vi "WAPIGetBoardType.vi"(9 "error in (no error)":errorcluster) -> (2 "Board Type":u32, 6 "error out":errorcluster)   [LabVIEW 2009]
uses:
  win50032.dll
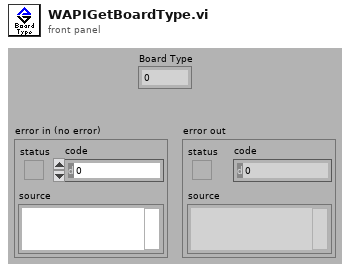
[diagram p1: front panel]
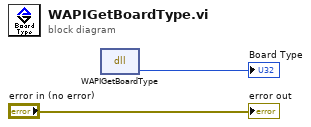
[diagram p0: block diagram]
diagram:
  n1 = dll-call lib="Win50032.dll" fn="WAPIGetBoardType" label="WAPIAerOpen"() -> ("return type"=→"Board Type":u32)  [unwired: 3 in, 2 out]
  "error out" <- "error in (no error)"
